vi "PopulateRings.vi"(8 "ErrorArray In":errorcluster[](array[cluster]), 10 "RelativePathToIniArray":string[](array[string])=["..\\..\\..\\Modules\\EventPlugins", "..\\..\\..\\Modules\\PmuImpairPlugins", "..\\..\\..\\Modules\\FlagImpairplugins", "..\\..\\..\\Modules\\NetworkImpairmentPlugins", "..\\..\\..\\Modules\\OutputToFilePlugins", "..\\..\\..\\Modules\\AppPlugins"], 11 "RingRefArray":refnum<vi>[](array[refnum])) -> (0 "ErrorArray Out":errorcluster[](array[cluster]), 2 "INIFilePathsArray":path[][](array[path]))   [LabVIEW 2014, in "Ini_lib.lvlib"]
uses:
  Ini_lib.lvlib
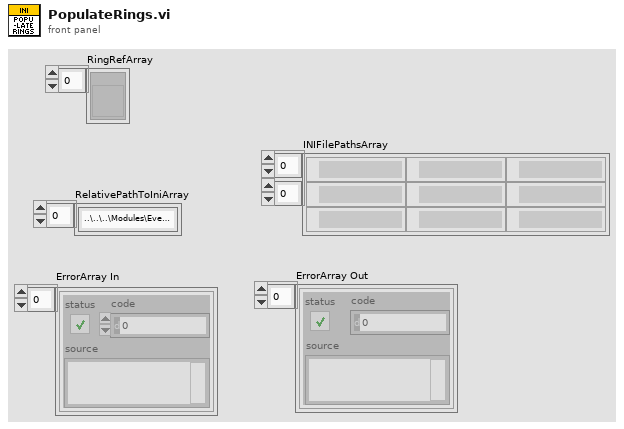
[diagram p1: front panel]
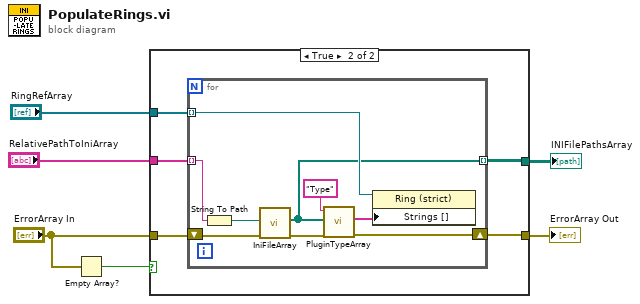
[diagram p0: block diagram]
diagram:
  n1 = Empty Array?(array="ErrorArray In") -> (empty?=w6:bool)
  n2 = case shown="True" w6 {
    tunnel: "ErrorArray In" -> [w7 w12]
    tunnel: [w7 w11] -> w4
    tunnel: "RingRefArray" -> [_ w10]
    tunnel: "RelativePathToIniArray" -> [_ w9]
    tunnel: [_ w8] -> w1
    frame False {
    }
    frame True {
      n3 = for {
        tunnel: w9 -> [w21] mode=indexing
        tunnel: w10 -> [w17] mode=indexing
        tunnel: [w13] -> w8 mode=indexing
        shift-right: [w14] -> w11
        shift-left: w12 -> [w15]
        n4 = String To Path(string=w21) -> (path=w20:path)
        n5 = call "IniFileArray.vi"("ErrorArray In"=w15, "Relative Path to Plugins"=w20) -> ("ErrorArray Out"=w18:errorcluster[], "INIFilePaths"=w13:path[])  [unwired: 8 in]
        n6 = call "PluginTypeArray.vi"("ErrorArray Out in"=w18, "INIFilePaths"=w13, "section"="Type") -> ("ErrorArray Out out"=w14:errorcluster[], "PluginTypes"=w16:string[])  [unwired: 6 in, 1 out]
        n7 = property class="Ring (strict)"(reference=w17, "Strings []"=w16) -> ()  [unwired: 1 in, 2 out]
      }
    }
  }
  "ErrorArray Out" <- w4
  "INIFilePathsArray" <- w1
